vi "Get Mapped Memory Access Information.vi"   [LabVIEW 2020, in "image.lvlib"]
doc: "Copy a LabVIEW Pixmap Image to an ARGB or Greyscale image with the option to generate a mask from the mask data in the Pixmap.\n\nOnly 8, 24 and 32-bit image depths are supported."
uses:
  image.lvlib
  Mapped Memory Access Image ARGB/Mapped Memory Access Image ARGB.lvclass
  Mapped Memory Access Image Greyscale/Mapped Memory Access Image Greyscale.lvclass
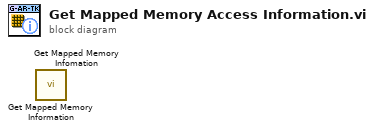
[diagram p0: block diagram]
diagram:
  n1 = call "Get Mapped Memory Information.vi"() -> ()  [unwired: 1 in, 1 out]
  n2 = call "Get Mapped Memory Infomation.vi"() -> ()  [unwired: 1 in, 1 out]
